vi "RSZVB Get Output Port Bits.vi"(8 "error in (no error)":errorcluster {"code" format="%.0x"}, 9 "Output Port (A)":i32(ring) items=["A", "B"], 11 "VISA session":refnum<visa-resource-name>) -> (0 "error out":errorcluster {"code" format="%.0x"}, 2 "Port Bits":i32, 3 "dup VISA session":refnum<visa-resource-name>)   [LabVIEW 2011]
doc: "This VI queries a channel-dependent bit pattern to the output ports A or B of the Universal Interface (option R&S ZVAB-B14). The channel bits are combined with the (static) output bits defined via CONTrol:HANDler:A|B[:DATA] using a logical \"or\" operation. The channel bits must be defined while the channel is active (CONTrol:NSELect <Ch>); the corresponding signals will be in effect while the channel is measured (dynamic output signals).\n\nRemote-control command(s):\nCONTrol:AUXiliary:<A|B>[:DATA]?"
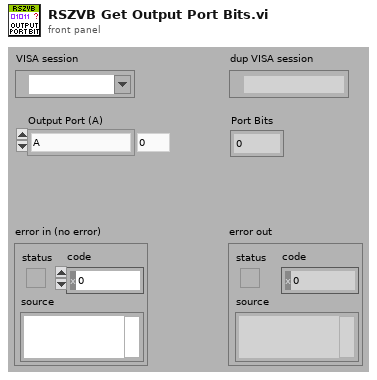
[diagram p1: front panel]
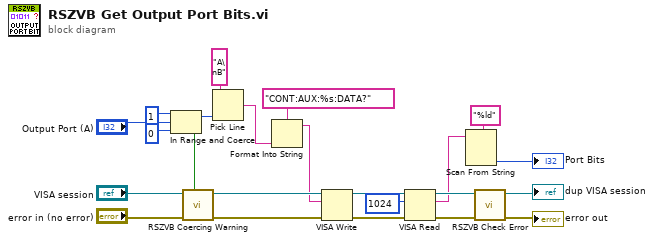
[diagram p0: block diagram]
diagram:
  n1 = In Range and Coerce(upper limit=1, x="Output Port (A)", lower limit=0) -> (coerced(x)=w6:i32, In Range?=w7:bool)
  n2 = call "RSZVB Coercing Warning.vi"("In Range?"=w7, "error in (no error)"="error in (no error)", "VISA session"="VISA session") -> ("error out"=w13:errorcluster, "dup VISA session"=w12:refnum<visa-resource-name>)  [unwired: 7 in]
  n3 = Pick Line(multi-line string="A\nB", line index=w6) -> (output string=w5:string)  [unwired: 1 in]
  n4 = Format Into String(format string="CONT:AUX:%s:DATA?", w5) -> (resulting string=w9:string)  [unwired: 2 in, 1 out]
  n5 = VISA Write(VISA resource name=w12, write buffer=w9, error in (no error)=w13) -> (VISA resource name out=w21:refnum<visa-resource-name>, error out=w23:errorcluster)  [unwired: 1 out]
  n6 = VISA Read(VISA resource name=w21, byte count=u32 1024 ("byte count (0)"), error in (no error)=w23) -> (VISA resource name out=w20:refnum<visa-resource-name>, read buffer=w2:string, error out=w19:errorcluster)  [unwired: 1 out]
  n7 = Scan From String(format string="%ld", input string=w2) -> (output 1=→"Port Bits":i32)  [unwired: 3 in, 3 out]
  n8 = call "RSZVB Check Error.vi"("error in (no error)"=w19, "VISA session"=w20) -> ("error out"=→"error out":errorcluster, "dup VISA session"=→"dup VISA session":refnum<visa-resource-name>)  [unwired: 8 in]
